vi "Define_Indicies_(101-11)_of_Affected_Tracks-1.vi"(4 "error IN":errorcluster, 5 "[IN] Subtracks":T2(array[cluster]), 6 "[IN] Indicies of sub\ntracks for transforma\ntion (resolving)":i32[](array[numeric]), 7 "[IN] Still connected\ntracks in group":T1) -> (0 "error OUT":errorcluster, 2 "[OUT] Indicies for Tr-\nack Reconstruction":i32[](array[numeric]))   [LabVIEW 2013]
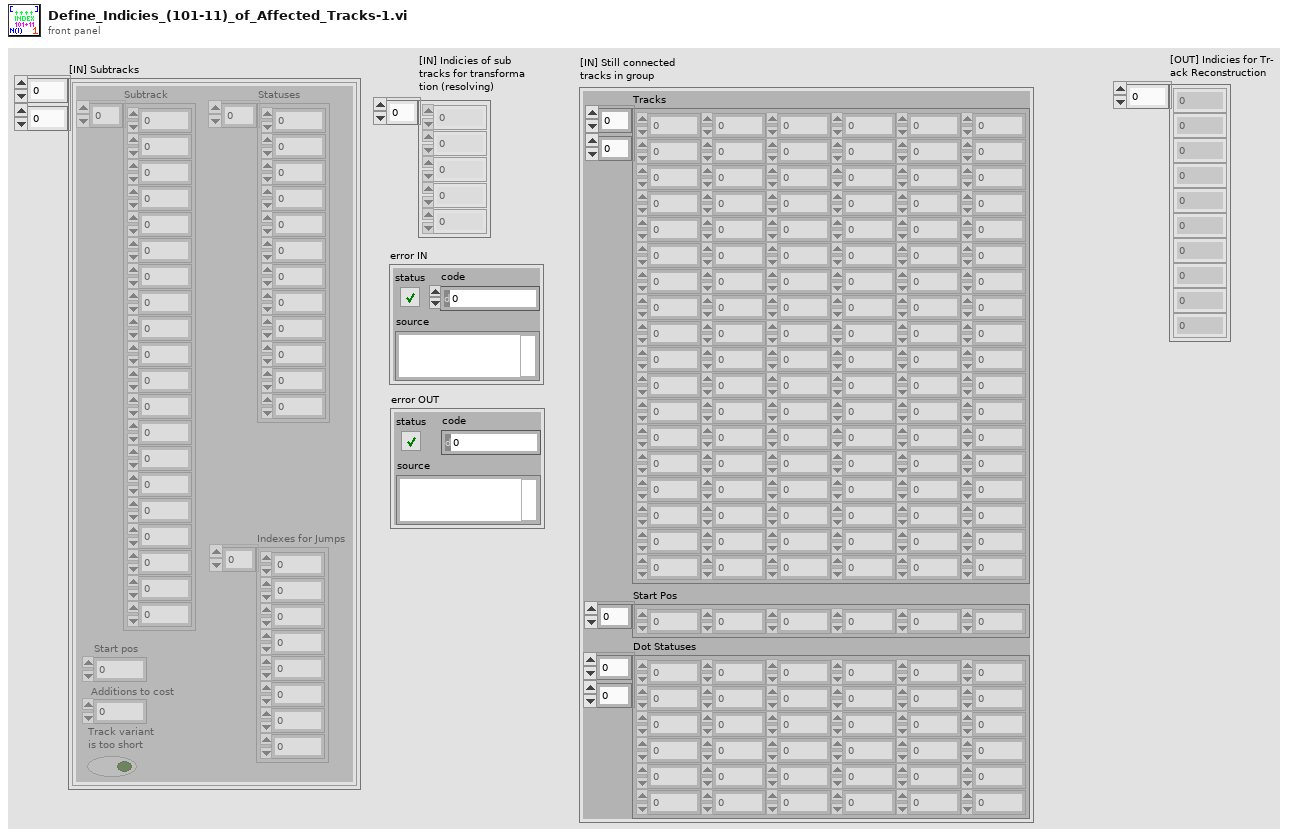
[diagram p1: front panel]
types:
  T1 = cluster{"Tracks":dbl[][], "Start Pos":i32[], "Dot Statuses":i16[][]}
  T2 = cluster{"Subtrack":dbl[], "Statuses":i16[], "Start pos":i32, "Additions to cost":i32, "Track variant \nis too short":bool, "Indexes for Jumps":i32[]}[][]
  T3 = cluster{"Subtrack":dbl[], "Statuses":i16[], "Start pos":i32, "Additions to cost":i32, "Track variant \nis too short":bool, "Indexes for Jumps":i32[]}[]
  T4 = cluster{"Subtrack":dbl[], "Statuses":i16[], "Start pos":i32, "Additions to cost":i32, "Track variant \nis too short":bool, "Indexes for Jumps":i32[]}
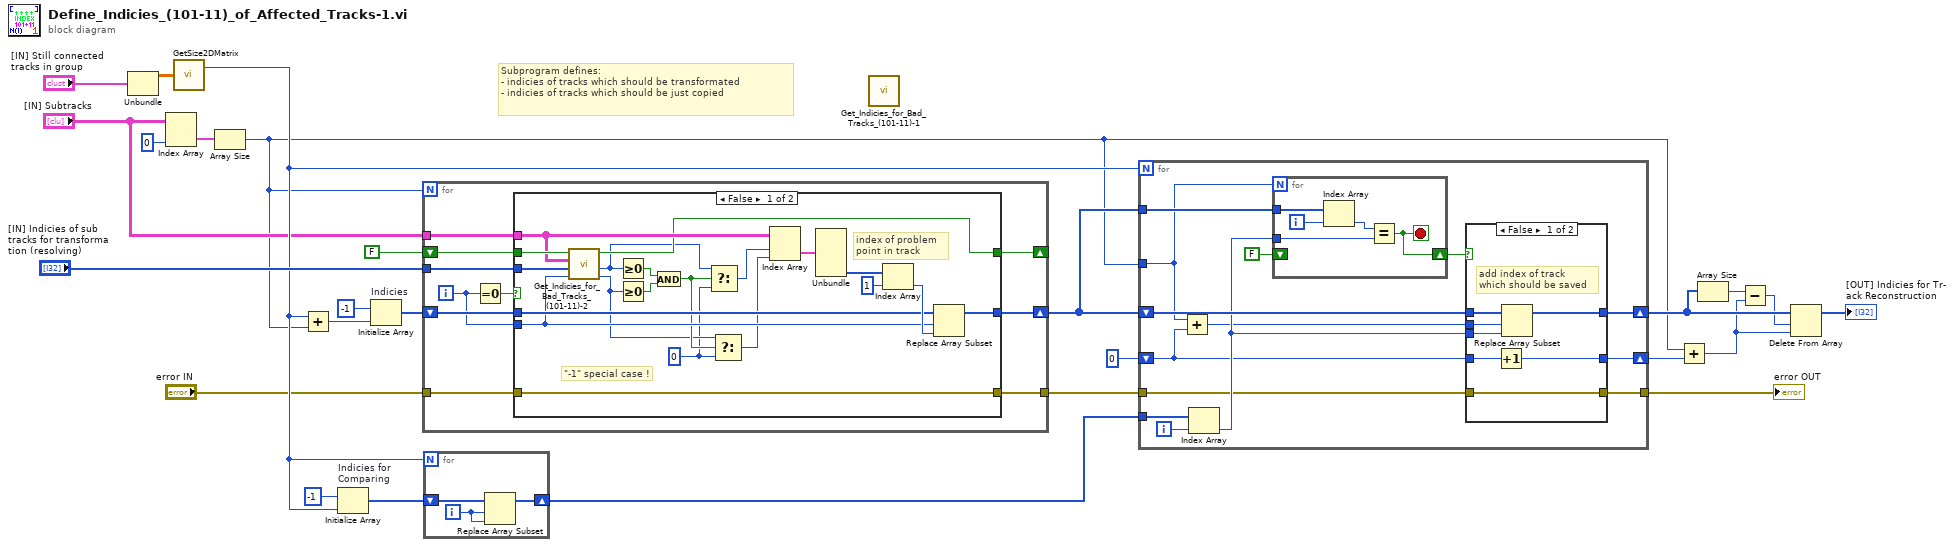
[diagram p0: block diagram]
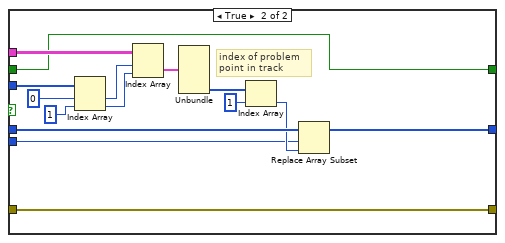
[diagram p3: hidden frame]
diagram:
  # "Subprogram defines:\n- indicies of tracks which should be transformated\n- indicies of tracks which should be just copied"
  n1 = Unbundle("[IN] Still connected\ntracks in group") -> ("Tracks"=w24:dbl[][])  [unwired: 2 out]
  n2 = Index Array(array="[IN] Subtracks", index (col)=0 ("disabled index (col)")) -> (element=w4:T3)  [unwired: 1 in]
  n3 = call "GetSize2DMatrix.vi"("Array IN (2D)"=w24) -> ("# Cols"=w17:i32)  [unwired: 1 out]
  n4 = Array Size(array=w4) -> (size(s)=w2:i32)
  n5 = Add(x=w17, y=w2) -> (x+y=w23:i32)
  n6 = Initialize Array "Indicies for \nComparing"(-1 ("# Cols"), w17) -> (w19:i32[])
  n7 = Initialize Array "Indicies"(-1 ("# Cols"), w23) -> (w21:i32[])
  n8 = for {
    N: w2 -> [_]
    tunnel: "[IN] Subtracks" -> [w36]
    tunnel: "[IN] Indicies of sub\ntracks for transforma\ntion (resolving)" -> [w30]
    shift-right: [w34] -> w16
    shift-left: w21 -> [w35]
    tunnel: "error IN" -> [w28]
    tunnel: [w27] -> w7
    shift-right: [w29] -> _
    shift-left: FALSE -> [w31]
    i -> [w33]
    n9 = Equal To 0?(x=w33) -> (x = 0?=w32:bool)
    n10 = case shown="False" w32 {
      tunnel: w36 -> [w46 w71]
      tunnel: w35 -> [w52 w67]
      tunnel: w33 -> [w47 w65]
      tunnel: [w51 w64] -> w34
      tunnel: w31 -> [w49 w58]
      tunnel: w30 -> [w48 w61]
      tunnel: [w45 w58] -> w29
      tunnel: w28 -> [w50 w57]
      tunnel: [w50 w57] -> w27
      frame False {
        w37 = 0 ("f")
        # "\"-1\" special case !"
        # "index of problem \npoint in track"
        n11 = call "Get_Indicies_for_Bad_Tracks_(101-11)-2.vi"("[IN] Current index"=w47, "[IN] Indicies of subtracks for \ntransformation (resolving)"=w48, "[IN] Subtracks"=w46, "[IN] Competed elonga\ntion is reconstructed?"=w49) -> ("[OUT] Column Number"=w40:i32, "[OUT] Row Number"=w42:i32, "[OUT] Competed elonga\ntion is reconstructed?"=w45:bool)  [unwired: 1 in]
        n12 = Greater Or Equal To 0?(x=w42) -> (x >= 0?=w44:bool)
        n13 = Greater Or Equal To 0?(x=w40) -> (x >= 0?=w43:bool)
        n14 = And(x=w44, y=w43) -> (x .and. y?=w41:bool)
        n15 = Select(t=w42, s=w41, f=w37) -> (s? t:f=w39:i32)
        n16 = Select(t=w40, s=w41, f=w37) -> (s? t:f=w38:i32)
        n17 = Index Array(array=w46, index (row)=w39, index (col)=w38) -> (element=w56:T4)
        n18 = Unbundle(w56) -> ("Indexes for Jumps"=w55:i32[])  [unwired: 5 out]
        n19 = Index Array(array=w55, index=1) -> (element=w53:i32)
        n20 = Replace Array Subset(array=w52, new element=w53, index=w47) -> (w51:i32[])
      }
      frame True {
        # "index of problem \npoint in track"
        n21 = Index Array(array=w61, index #1=0 ("index"), index #2=1 ("index")) -> (element #1=w60:i32, element #2=w59:i32)
        n22 = Index Array(array=w71, index (row)=w60, index (col)=w59) -> (element=w70:T4)
        n23 = Unbundle(w70) -> ("Indexes for Jumps"=w69:i32[])  [unwired: 5 out]
        n24 = Index Array(array=w69, index=1) -> (element=w66:i32)
        n25 = Replace Array Subset(array=w67, new element=w66, index=w65) -> (w64:i32[])
      }
    }
  }
  n26 = for {
    N: w17 -> [_]
    shift-right: [w72] -> w18
    shift-left: w19 -> [w74]
    i -> [w73]
    n27 = Replace Array Subset(array=w74, new element=w73, index=w73) -> (w72:i32[])
  }
  n28 = call "Get_Indicies_for_Bad_Tracks_(101-11)-1.vi"() -> ()  [unwired: 3 in, 3 out]
  n29 = for {
    N: w17 -> [_]
    tunnel: w2 -> [w80]
    shift-right: [w82] -> w13
    shift-left: w16 -> [w83]
    tunnel: w18 -> [w88]
    tunnel: w16 -> [w86]
    shift-right: [w77] -> w14
    shift-left: 0 -> [w78]
    tunnel: w7 -> [w76]
    tunnel: [w75] -> w6
    i -> [w87]
    n30 = Add(x=w80, y=w78) -> (x+y=w79:i32)
    n31 = Index Array(array=w88, index=w87) -> (element=w81:i32)
    n32 = for {
      N: w80 -> [_]
      tunnel: w86 -> [w103]
      tunnel: w81 -> [w100]
      shift-right: [w99] -> w84
      shift-left: FALSE -> [_]
      i -> [w102]
      stop <- w99 stop-if-true
      n33 = Index Array(array=w103, index=w102) -> (element=w101:i32)
      n34 = Equal?(x=w101, y=w100) -> (x = y?=w99:bool)
    }
    n35 = case shown="False" w84 {
      tunnel: w83 -> [w95 w98]
      tunnel: [w92 w98] -> w82
      tunnel: w81 -> [w94 _]
      tunnel: w79 -> [w93 _]
      tunnel: w78 -> [w91 w97]
      tunnel: [w90 w97] -> w77
      tunnel: w76 -> [w89 w96]
      tunnel: [w89 w96] -> w75
      frame False {
        # "add index of track\nwhich should be saved"
        n36 = Increment(x=w91) -> (x+1=w90:i32)
        n37 = Replace Array Subset(array=w95, new element=w94, index=w93) -> (w92:i32[])
      }
      frame True {
      }
    }
  }
  "error OUT" <- w6
  n38 = Add(x=w2, y=w14) -> (x+y=w11:i32)
  n39 = Array Size(array=w13) -> (size(s)=w12:i32)
  n40 = Subtract(x=w12, y=w11) -> (x-y=w10:i32)
  n41 = Delete From Array(array=w13, length=w10, index=w11) -> (array with subset deleted=→"[OUT] Indicies for Tr-\nack Reconstruction":i32[])  [unwired: 1 out]
